vi "GetMonitorDatav2.vi"(7 "LabVIEW Web Service Request":refnum<class "Web Request.lvclass">, 11 "Channel":i32) -> (3 "LVArray":dbl[][](array[numeric]))   [LabVIEW 2018]
uses:
  <vilib>/wsapi/Web Request.lvclass
  CAEN globals.vi
  <userlib>/_OpenG.lib/array/array.llb/Search 1D Array (I32)__ogtk.vi
  <vilib>/Analysis/Matrix/Numeric/Conversions/Matrix To Array - RM.vi
  <vilib>/Analysis/Matrix/NI_Matrix.lvlib
panel:
  out "error out":errorcluster
  in  "error in (no error)":errorcluster
  # "Use the Web Service Request input terminal to call the VIs on the Web Services palette. Do not remove it from the connector pane unless you don't need access to the palette."
  # "Each additional control wired to the connector pane will be available as an input in the URL. To include an indicator in terminal-mode output (the default setting), it must also be wired to the connector pane."
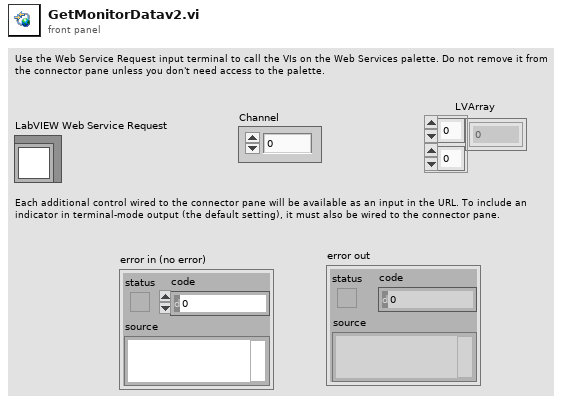
[diagram p1: front panel]
types:
  T1 = typedef "NI_Matrix.lvlib/RealMatrix.ctl" = dbl[][]
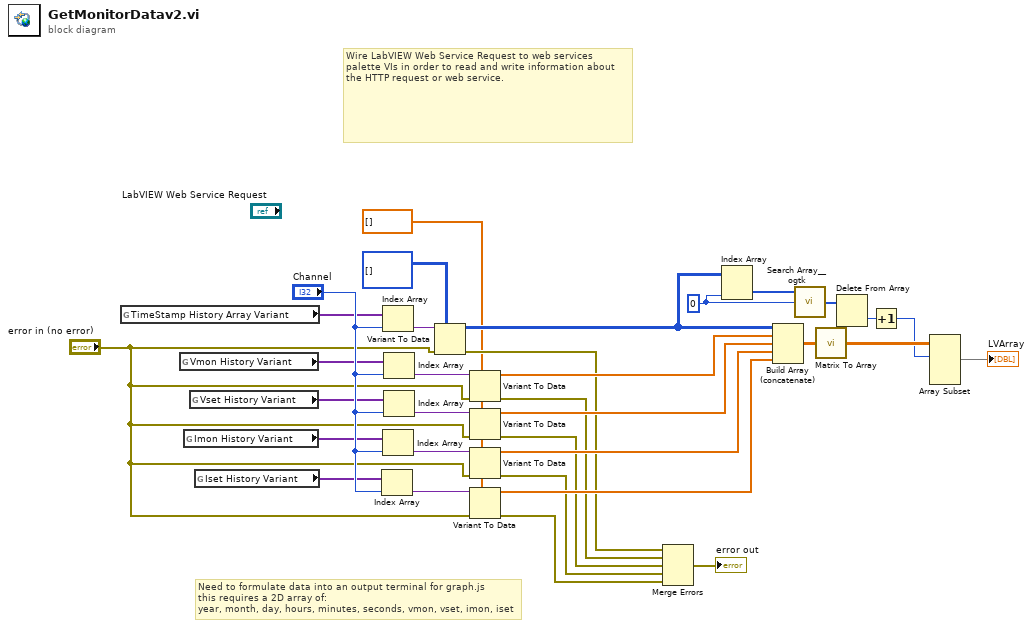
[diagram p0: block diagram]
diagram:
  w7 = dbl[] [] ("Value")
  w26 = 0 ("disabled index (col)")
  # "Need to formulate data into an output terminal for graph.js\nthis requires a 2D array of:\nyear, month, day, hours, minutes, seconds, vmon, vset, imon, iset"
  # "Wire LabVIEW Web Service Request to web services palette VIs in order to read and write information about the HTTP request or web service."
  n1 = global read "CAEN globals.vi" "TimeStamp History Array Variant"() -> (w6:variant[])
  n2 = global read "CAEN globals.vi" "Vmon History Variant"() -> (w2:variant[])
  n3 = global read "CAEN globals.vi" "Imon History Variant"() -> (w4:variant[])
  n4 = global read "CAEN globals.vi" "Vset History Variant"() -> (w3:variant[])
  n5 = global read "CAEN globals.vi" "Iset History Variant"() -> (w5:variant[])
  n6 = Index Array(array=w5, index="Channel") -> (element=w14:variant)
  n7 = Index Array(array=w6, index="Channel") -> (element=w23:variant)
  n8 = Index Array(array=w4, index="Channel") -> (element=w16:variant)
  n9 = Index Array(array=w2, index="Channel") -> (element=w20:variant)
  n10 = Index Array(array=w3, index="Channel") -> (element=w18:variant)
  n11 = Variant To Data(error in="error in (no error)", type=i32[][] [] ("Value"), Variant=w23) -> (data=w21:i32[][], error out=w12:errorcluster)
  n12 = Variant To Data(error in="error in (no error)", type=w7, Variant=w20) -> (data=w19:dbl[], error out=w11:errorcluster)
  n13 = Variant To Data(error in="error in (no error)", type=w7, Variant=w18) -> (data=w17:dbl[], error out=w10:errorcluster)
  n14 = Variant To Data(error in="error in (no error)", type=w7, Variant=w16) -> (data=w15:dbl[], error out=w9:errorcluster)
  n15 = Variant To Data(error in="error in (no error)", type=w7, Variant=w14) -> (data=w13:dbl[], error out=w8:errorcluster)
  n16 = Merge Errors(w12, w11, w10, w9, w8) -> (→"error out":errorcluster)
  n17 = Index Array(array=w21, index (col)=w26) -> (element=w27:i32[])  [unwired: 1 in]
  n18 = Build Array (concatenate)(w21, w19, w17, w15, w13) -> (w33:T1)
  n19 = call-poly <userlib>:"Search Array__ogtk.vi"("Array"=w27, "Element Data"=w26) -> ("Indices of Elements"=w29:i32[])  [unwired: 7 in]
  n20 = call-poly <vilib>:"Matrix To Array.vi"("Real Matrix"=w33) -> ("Real 2D Array"=w31:dbl[][])
  n21 = Delete From Array(array=w29) -> (deleted portion=w28:i32)  [unwired: 2 in, 1 out]
  n22 = Increment(x=w28) -> (x+1=w25:i32)
  n23 = Array Subset(array=w31, index (row)=w25) -> (→"LVArray":dbl[][])  [unwired: 3 in]
